vi "Subscriber.vi"(8 "error in":errorcluster {"code" format="Error %.0f"}) -> (0 "error out":errorcluster)   [LabVIEW 2024]
uses:
  NATS Subscription/NATS Subscription.lvclass
  NATS Subscription/NATS Subscription.lvclass/NATS Subscription.ctl
  NATS Client/NATS Client.lvclass/NATS Client.ctl
  NATS Subscription/get subject.vi
  <vilib>/NATS/NATS Core/VIs/NATS CLOSE.vi
  NATS Client/get async stop notifier.vi
  NATS Client/Get Connection DVR.vi
  NATS Client/get subscriptions queue.vi
  NATS Client/Get subscription map.vi
  NATS Client/Get error queue.vi
  NATS Client/NATS Client.lvclass
panel:
  out "Active Subscriptions":T1(array[cluster])
  out "Server Connected":bool
  out "Payload":string
  out "Received":timestamp format="%<%.0X %x>T"
  in  "Read":bool
  in  "Unsubscribe":bool
  out "loop error":errorcluster
  in  "Subscribe":bool
  in  "Subject":string="data.hello_world"
  # "Subject Wildcards\nThe first wildcard is * which will match a single token. \n\nNote that * can not match a substring within a token time.New*.east.\n\nMatching multiple tokens\nThe second wildcard is > which will match one or more tokens,\nand can only appear at the end of the subject."
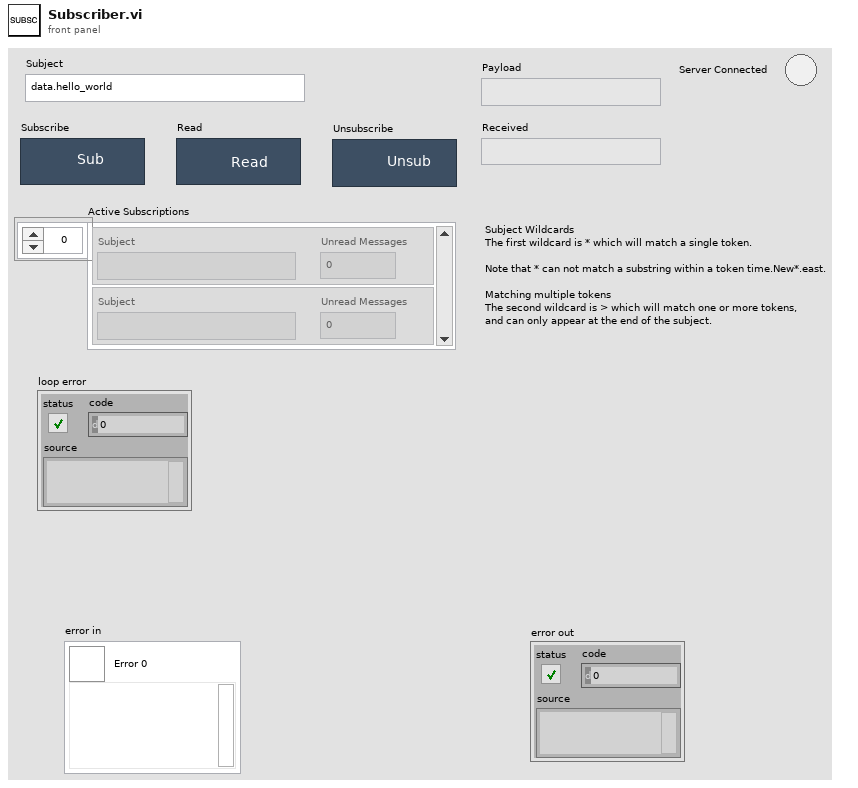
[diagram p1: front panel]
types:
  T1 = cluster{"Subject":string, "Unread Messages":i32}[]
  T2 = map{string, refnum<class "NATS Subscription.lvclass">}
  T3 = typedef "NATS Core.lvlib/nats message.ctl" = cluster{"subject":string, "payload":string, "sub id":string, "reply-to":string, "headers":string, "type":T4, "received":timestamp}
  T4 = typedef "NATS Core.lvlib/msg type.ctl" = enum16{"Undefined", "MSG", "HMSG", "+OK", "PING", "PONG", "-ERR", "INFO"}
  T5 = cluster{"Properties:subject":string, "# elements in queue":i32}
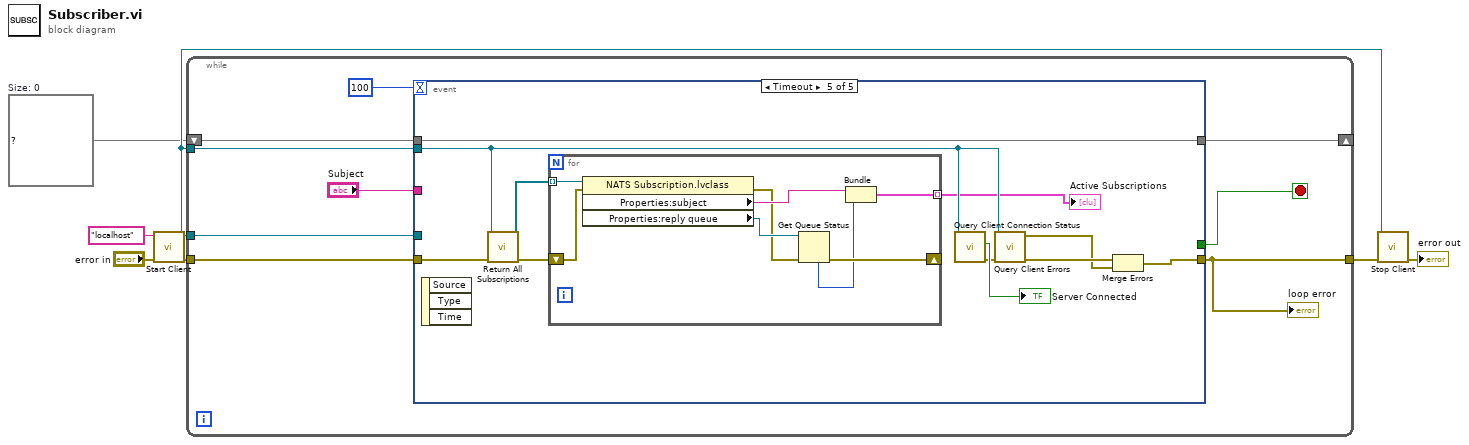
[diagram p0: block diagram]
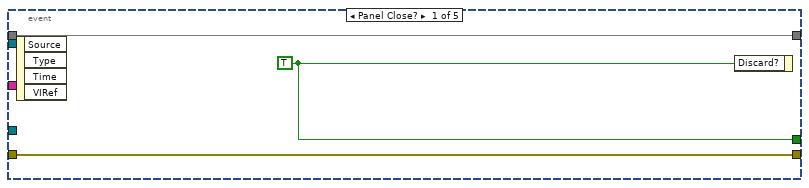
[diagram p2: hidden frame]
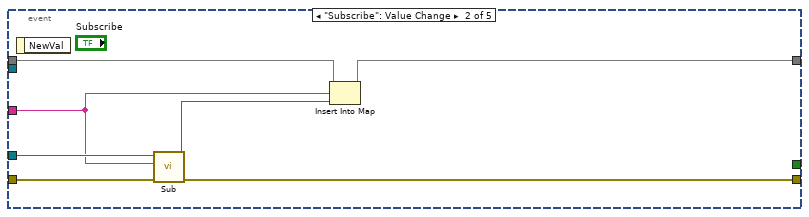
[diagram p3: hidden frame]
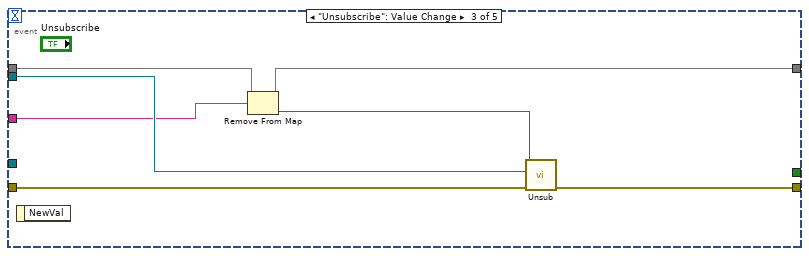
[diagram p4: hidden frame]
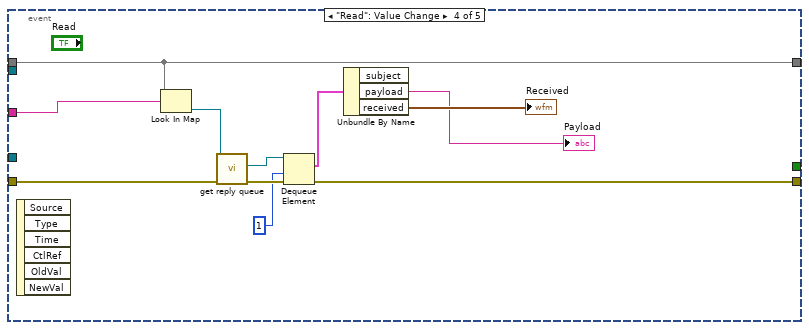
[diagram p5: hidden frame]
diagram:
  w2 = T2 {}  # Size: 0
  n1 = call "Start Client.vi"("error in"="error in", "address"="localhost") -> ("error out"=w7:errorcluster, "NATS Client out"=w4:refnum<class "NATS Client.lvclass">)  [unwired: 8 in]
  n2 = while {
    tunnel: w4 -> [w14]
    tunnel: w4 -> [w9]
    shift-right: [w13] -> _
    shift-left: w2 -> [w12]
    tunnel: w7 -> [w15]
    tunnel: [w8] -> w5
    stop <- w16 stop-if-true
    n3 = event shown="[4] Timeout" {
      selector: _ -> [_ _ _ _ _]
      dyn-events: _ -> [_ _ _ _ _]
      timeout: 100 -> [_ _ _ _ _]
      tunnel: [w19 _ _ _ _] -> w16
      tunnel: w15 -> [w18 w25 w31 w44 w49]
      tunnel: [w18 w24 w32 w34 w52] -> w8
      tunnel: w14 -> [_ w26 _ _ _]
      tunnel: w9 -> [_ _ w33 _ w48]
      tunnel: [w17 w20 w28 w37 w51] -> w13
      tunnel: w12 -> [w17 w21 w27 w37 w51]
      tunnel: "Subject" -> [_ w23 w30 w43 _]
      event Panel Close? {
        w19 = TRUE ("Discard?")
        n4 = event-data() -> ()  [unwired: 1 in, 4 out]
        n5 = event-data("Discard?"=w19) -> ()  [unwired: 1 in, 1 out]
      }
      event "Subscribe": Value Change {
        n6 = event-data() -> ()  [unwired: 1 in, 1 out]
        n7 = call "Sub.vi"("error in"=w25, "subject"=w23, "NATS Client"=w26) -> ("error out"=w24:errorcluster, "NATS Subscription"=w22:refnum<class "NATS Subscription.lvclass">)  [unwired: 7 in]
        n8 = Insert Into Map(map in=w21, key=w23, value=w22) -> (map out=w20:T2)  [unwired: 2 out]
      }
      event "Unsubscribe": Value Change {
        n9 = event-data() -> ()  [unwired: 1 in, 1 out]
        n10 = Remove From Map(10:w30, 11:w27) -> (1:w29:refnum<class "NATS Subscription.lvclass">, 3:w28:T2)  [unwired: 1 out]
        n11 = call "Unsub.vi"("error in"=w31, "NATS Client"=w33, "NATS Subscription"=w29) -> ("error out"=w32:errorcluster)  [unwired: 7 in, 1 out]
      }
      event "Read": Value Change {
        n12 = event-data() -> ()  [unwired: 1 in, 6 out]
        n13 = Look In Map(map=w37, key=w43) -> (value=w42:refnum<class "NATS Subscription.lvclass">)  [unwired: 1 in, 1 out]
        n14 = call "get reply queue.vi"("error in"=w44, "NATS Subscription in"=w42) -> ("error out"=w41:errorcluster, "reply queue"=w35:refnum<queue>)  [unwired: 7 in, 1 out]
        n15 = Dequeue Element(queue=w35, timeout in ms (-1)=1, error in (no error)=w41) -> (element=w40:T3, error out=w34:errorcluster)  [unwired: 2 out]
        n16 = Unbundle By Name(w40) -> ("payload"=→"Payload":string, "received"=→"Received":timestamp)  [unwired: 1 out]
      }
      event Timeout {
        n17 = event-data() -> ()  [unwired: 1 in, 3 out]
        n18 = call "Return All Subscriptions.vi"("error in"=w49, "NATS Client"=w48) -> ("error out"=w47:errorcluster, "Subscriptions"=w50:refnum<class "NATS Subscription.lvclass">[])  [unwired: 8 in]
        n19 = for {
          tunnel: w50 -> [w63] mode=indexing
          shift-right: [w61] -> _
          shift-left: w47 -> [w57]
          tunnel: [w58] -> w45 mode=indexing
          n20 = property class="NATS Subscription.lvclass"(reference=w63, error in=w57) -> (error out=w56:errorcluster, "Properties:subject"=w59:string, "Properties:reply queue"=w62:refnum<queue>)  [unwired: 1 out]
          n21 = Get Queue Status(queue=w62, error in (no error)=w56) -> (error out=w61:errorcluster, # elements in queue=w60:i32)  [unwired: 1 in, 6 out]
          n22 = Bundle("Properties:subject"=w59, "# elements in queue"=w60) -> (w58:T5)  [unwired: 1 in]
        }
        "Active Subscriptions" <- w45
        n23 = call "Query Client Connection Status.vi"("NATS Client in"=w48) -> ("error out"=w54:errorcluster, "Connected"=→"Server Connected":bool)  [unwired: 9 in]
        n24 = call "Query Client Errors.vi"("error in"=w54, "NATS Client"=w48) -> ("error out"=w53:errorcluster, "errors"=w46:errorcluster[])  [unwired: 8 in]
        n25 = Merge Errors(w53, w46) -> (w52:errorcluster)
      }
    }
    "loop error" <- w8
  }
  n26 = call "Stop Client.vi"("error in"=w5, "NATS Client"=w4) -> ("error out"=→"error out":errorcluster)  [unwired: 9 in]
